vi "ParseSysexAnalogMappingResponse.vi"(8 "error in":errorcluster, 10 "Sysex Message":u8[](array[numeric]) format="%x") -> (0 "error out":errorcluster, 1 "IsValidSysex":bool, 2 "AnalogChannels":u8[](array[numeric]))   [LabVIEW 2020]
doc: "Parse a message according to the Firmata Protocol Requirements. \n- https://github.com/firmata/protocol\n- https://github.com/firmata/protocol/blob/master/protocol.md"
uses:
  Controls/FirmataProtocolConstants.ctl
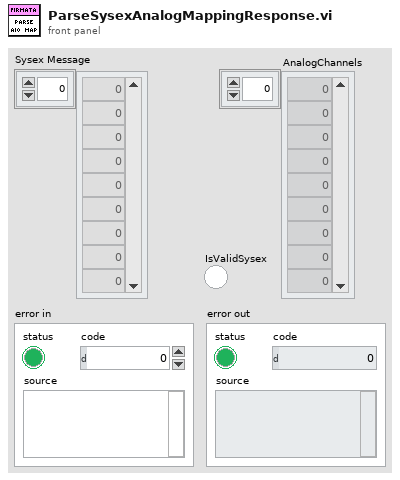
[diagram p1: front panel]
types:
  T1 = typedef "FirmataProtocolConstants.ctl" = u16
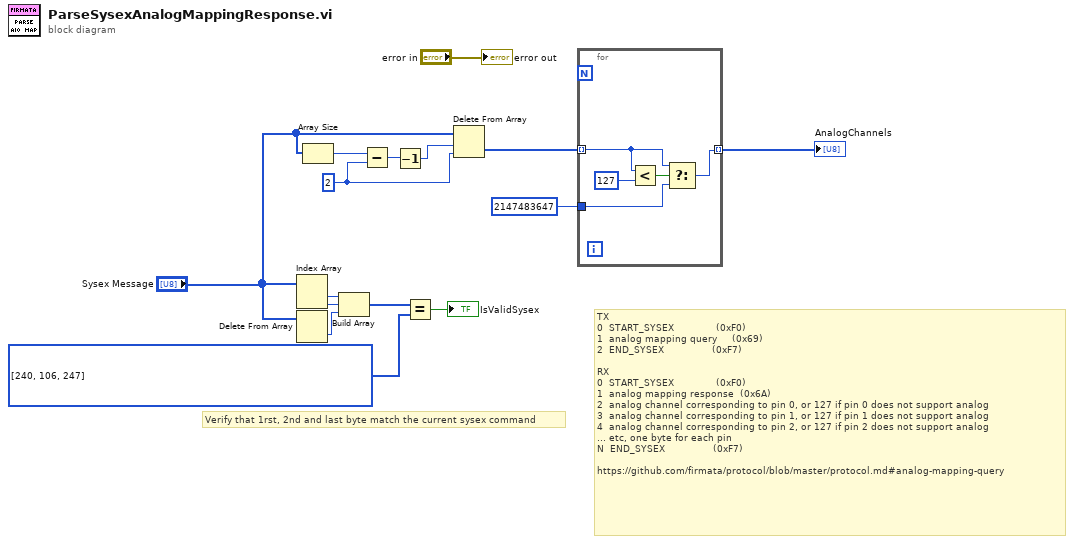
[diagram p0: block diagram]
diagram:
  w5 = T1[] [240, 106, 247] items=["ANALOG_IO_MESSAGE"=224, "DIGITAL_IO_MESSAGE"=144, "REPORT_ANALOG_PIN"=192, "REPORT_DIGITAL_PORT"=208, "START_SYSEX"=240, "END_SYSEX"=247, "SET_PIN_MODE"=244, "SET_DIGITAL_PIN_VALUE"=245, "PROTOCOL_VERSION"=249, "SYSTEM_RESET"=255, "SYSEX.EXTENDED_ID"=0, "SYSEX.RESERVED_USER_COMMANDs"=1, "SYSEX.ANALOG_MAPPING_QUERY"=105, "SYSEX.ANALOG_MAPPING_RESPONSE"=106, "SYSEX.CAPABILITY_QUERY"=107, "SYSEX.CAPABILITY_RESPONSE"=108, "SYSEX.PIN_STATE_QUERY"=109, "SYSEX.PIN_STATE_RESPONSE"=110, "SYSEX.REPORT_FIRMWARE"=121, "SYSEX.EXTENDED_ANALOG"=111, "SYSEX.STRING_DATA"=113, "SYSEX.REALTIME"=127, "SYSEX.NON_REALTIME"=126, "SYSEX.SAMPLING_INTERVAL"=122, "FEATURES.SYSEX.I2C_READ_WRITE"=118, "FEATURES.SYSEX.I2C_REPLY"=119, "FEATURES.SYSEX.I2C_CONFIG"=120]
  w8 = 2 ("index")
  # "Verify that 1rst, 2nd and last byte match the current sysex command"
  # "TX\n0  START_SYSEX              (0xF0)\n1  analog mapping query     (0x69)\n2  END_SYSEX                (0xF7)\n\nRX\n0  START_SYSEX              (0xF0)\n1  analog mapping response  (0x6A)\n2  analog channel corresponding to pin 0, or 127 if pin 0 does not support analog\n3  analog channel corresponding to pin 1, or 127 if pin 1 does not support analog\n4  analog channel corresponding to pin 2, or 127 if pin 2 does not support analog\n... etc, one byte for each pin\nN  END_SYSEX                (0xF7)\n\nhttps://github.com/firmata/protocol/blob/master/protocol.md#analog-mapping-query"
  n1 = Index Array(array="Sysex Message") -> (element #1=w15:u8, element #2=w13:u8)  [unwired: 2 in]
  n2 = Delete From Array(array="Sysex Message") -> (deleted portion=w14:u8)  [unwired: 2 in, 1 out]
  n3 = Array Size(array="Sysex Message") -> (size(s)=w9:i32)
  n4 = Build Array(w15, w13, w14) -> (w12:u8[])
  n5 = Subtract(x=w9, y=w8) -> (x-y=w7:i32)
  n6 = Decrement(x=w7) -> (x-1=w6:i32)
  n7 = Equal?(x=w12, y=w5) -> (x = y?=→"IsValidSysex":bool)
  n8 = Delete From Array(array="Sysex Message", length=w6, index=w8) -> (deleted portion=w2:u8[])  [unwired: 1 out]
  n9 = for {
    tunnel: [w17] -> w3 mode=indexing
    tunnel: w2 -> [w18] mode=indexing
    tunnel: 2147483647 ("y") -> [w16]
    n10 = Less?(x=w18, y=u8 127) -> (x < y?=w19:bool)
    n11 = Select(t=w18, s=w19, f=w16) -> (s? t:f=w17:i32)
  }
  "AnalogChannels" <- w3
  "error out" <- "error in"
